vi "TCP Parse NART Response.vi"(5 "Response":T2, 7 "Response Template":T2, 11 "error in":errorcluster) -> (8 "TX Response":T1, 15 "error out":errorcluster)   [LabVIEW 2012]
uses:
  Controls/QCA NART Message.ctl
  Controls/QCA NART Response Type.ctl
  Controls/QCA NART Response SubType.ctl
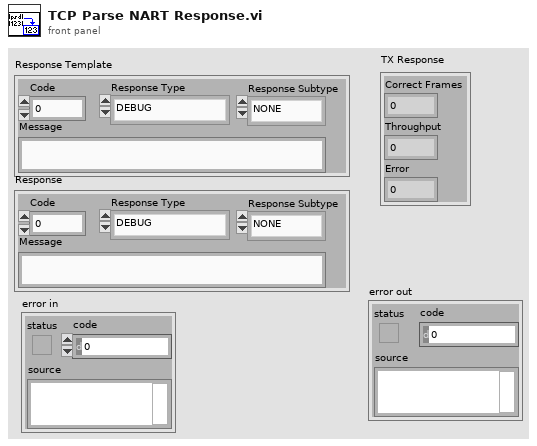
[diagram p1: front panel]
types:
  T1 = cluster{"Correct Frames":i32, "Throughput":i32, "Error":i32}
  T2 = typedef "QCA NART Message.ctl" = cluster{"Code":dbl, "Response Type":T3, "Response Subtype":T4, "Message":string}
  T3 = typedef "QCA NART Response Type.ctl" = enum16{"DEBUG", "CONTROL", "INFO", "WARNING", "ERROR", "NONE"}
  T4 = typedef "QCA NART Response SubType.ctl" = enum16{"NONE", "OK", "ON", "OFF", "BEGIN", "DONE"}
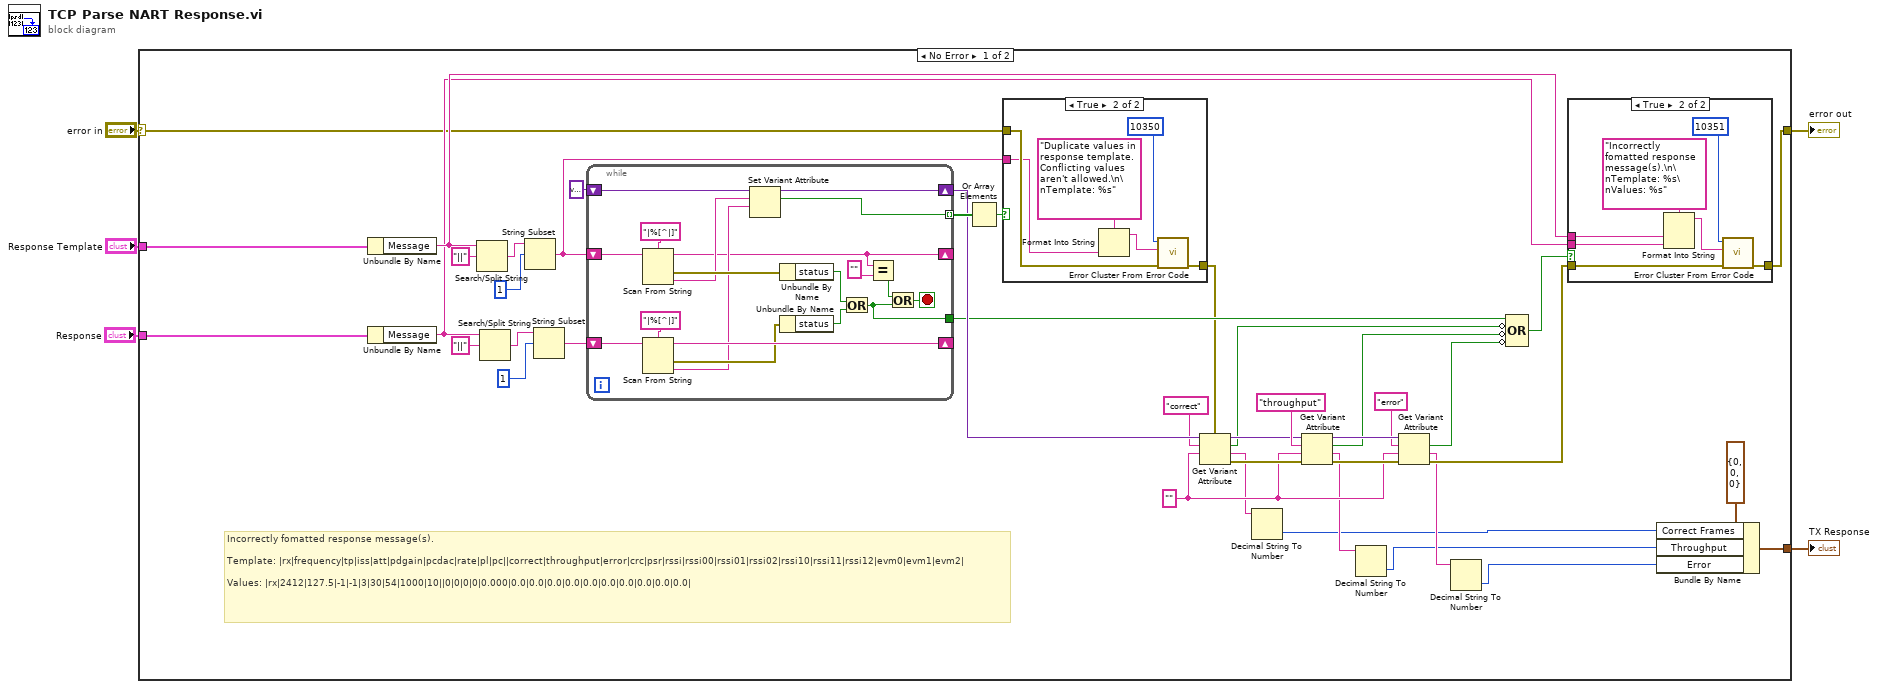
[diagram p0: block diagram]
diagram:
  n1 = case shown="No Error" "error in" {
    selector: "error in" -> [w6 w81]
    tunnel: [w13 w81] -> w2
    tunnel: "Response" -> [w44 _]
    tunnel: "Response Template" -> [w43 _]
    tunnel: [w45 _] -> w1
    frame No Error {
      w21 = "" ("name")
      # "Incorrectly fomatted response message(s).\n\nTemplate: |rx|frequency|tp|iss|att|pdgain|pcdac|rate|pl|pc||correct|throughput|error|crc|psr|rssi|rssi00|rssi01|rssi02|rssi10|rssi11|rssi12|evm0|evm1|evm2|\n\nValues: |rx|2412|127.5|-1|-1|3|30|54|1000|10||0|0|0|0|0.000|0.0|0.0|0.0|0.0|0.0|0.0|0.0|0.0|0.0|0.0|"
      n2 = Unbundle By Name(w43) -> ("Message"=w31:string)
      n3 = Unbundle By Name(w44) -> ("Message"=w30:string)
      n4 = Search/Split String(string=w31, search string/char (-)="||") -> (match + rest of string=w40:string)  [unwired: 1 in, 2 out]
      n5 = Search/Split String(string=w30, search string/char (-)="||") -> (match + rest of string=w39:string)  [unwired: 1 in, 2 out]
      n6 = String Subset(string=w40, offset (0)=1) -> (substring=w32:string)  [unwired: 1 in]
      n7 = String Subset(string=w39, offset (0)=1) -> (substring=w36:string)  [unwired: 1 in]
      n8 = while {
        shift-right: [w63] -> _
        shift-left: w32 -> [w80]
        shift-right: [w75] -> _
        shift-left: w36 -> [w76]
        tunnel: [w65] -> w16
        shift-right: [w68] -> w29
        shift-left: variant ("variant out") -> [w73]
        tunnel: [w67] -> w34 mode=indexing
        stop <- w66 stop-if-true
        n9 = Scan From String(format string="|%[^|]", input string=w80) -> (remaining string=w63:string, error out=w78:errorcluster, output 1=w70:string)  [unwired: 3 in, 1 out]
        n10 = Scan From String(format string="|%[^|]", input string=w76) -> (remaining string=w75:string, error out=w71:errorcluster, output 1=w69:string)  [unwired: 3 in, 1 out]
        n11 = Set Variant Attribute(Variant=w73, name=w70, value=w69) -> (Variant out=w68:variant, replaced=w67:bool)  [unwired: 1 in, 1 out]
        n12 = Unbundle By Name(w78) -> ("status"=w74:bool)
        n13 = Unbundle By Name(w71) -> ("status"=w72:bool)
        n14 = Or(x=w74, y=w72) -> (x .or. y?=w65:bool)
        n15 = Equal?(x=w63, y="" ("x")) -> (x = y?=w62:bool)
        n16 = Or(x=w62, y=w65) -> (x .or. y?=w66:bool)
      }
      n17 = Or Array Elements(Boolean array=w34) -> (logical OR=w33:bool)
      n18 = case shown="True" w33 {
        tunnel: w6 -> [w55 w61]
        tunnel: [w55 w60] -> w15
        tunnel: w32 -> [_ w56]
        frame False {
        }
        frame True {
          n19 = Format Into String(format string="Duplicate values in response template. Conflicting values aren't allowed.\n\nTemplate: %s", w56) -> (resulting string=w58:string)  [unwired: 2 in, 1 out]
          n20 = call <vilib>:"Error Cluster From Error Code.vi"("error in (no error)"=w61, "error message (\"\")"=w58, "error code (0)"=10350) -> ("error out"=w60:errorcluster)  [unwired: 6 in]
        }
      }
      n21 = Get Variant Attribute(Variant=w29, name="correct", default value (empty Variant)=w21, error in=w15) -> (duplicate Variant=w24:variant, found=w18:bool, value=w17:string, error out=w27:errorcluster)
      n22 = Decimal String To Number(string=w17) -> (number=w9:i32)  [unwired: 2 in, 1 out]
      n23 = Get Variant Attribute(Variant=w24, name="throughput", default value (empty Variant)=w21, error in=w27) -> (duplicate Variant=w23:variant, found=w19:bool, value=w11:string, error out=w26:errorcluster)
      n24 = Decimal String To Number(string=w11) -> (number=w8:i32)  [unwired: 2 in, 1 out]
      n25 = Get Variant Attribute(Variant=w23, name="error", default value (empty Variant)=w21, error in=w26) -> (found=w20:bool, value=w10:string, error out=w14:errorcluster)  [unwired: 1 out]
      n26 = Decimal String To Number(string=w10) -> (number=w7:i32)  [unwired: 2 in, 1 out]
      n27 = Compound Arithmetic op=OR(w16, invert w18, invert w19, invert w20) -> (w12:bool)
      n28 = case shown="True" w12 {
        tunnel: w14 -> [w47 w54]
        tunnel: [w47 w53] -> w13
        tunnel: w31 -> [_ w49]
        tunnel: w30 -> [_ w48]
        frame False {
        }
        frame True {
          n29 = Format Into String(format string="Incorrectly fomatted response message(s).\n\nTemplate: %s\nValues: %s", w49, w48) -> (resulting string=w51:string)  [unwired: 2 in, 1 out]
          n30 = call <vilib>:"Error Cluster From Error Code.vi"("error in (no error)"=w54, "error message (\"\")"=w51, "error code (0)"=10351) -> ("error out"=w53:errorcluster)  [unwired: 6 in]
        }
      }
      n31 = Bundle By Name(cluster=T1 {"Correct Frames"=0, "Throughput"=0, "Error"=0} ("TX Response"), "Correct Frames"=w9, "Throughput"=w8, "Error"=w7) -> (w45:T1)
    }
    frame Error {
    }
  }
  "error out" <- w2
  "TX Response" <- w1
